vi "Update Palette with Legend.vi"(6 "Control Ref Queue":T1, 8 "error in (no error)":errorcluster, 11 "3D Plot.lvclass":refnum<class "3D Plot.lvclass">) -> (0 "error out":errorcluster, 1 "Ignore the size change?":bool, 3 "3D Plot.lvclass out":refnum<class "3D Plot.lvclass">)   [LabVIEW 2017, in "3D Plot.lvclass"]
uses:
  <vilib>/Math Plots/3D Math Plots/3D Plot/3D Plot/3D Plot.lvclass
  <vilib>/Math Plots/3D Math Plots/3D Plot/Action String/3DMathPlot Ctrl Act Queue.ctl
  <vilib>/Math Plots/3D Math Plots/3D Plot/Action String/3DMathPlot Ctrl Act Cluster.ctl
  <vilib>/Math Plots/3D Math Plots/3D Plot/Action String/3DMathPlot State Class.ctl
  <vilib>/Math Plots/3D Math Plots/3D Plot/3D Plot/3D Plot.lvclass/3D Plot.ctl
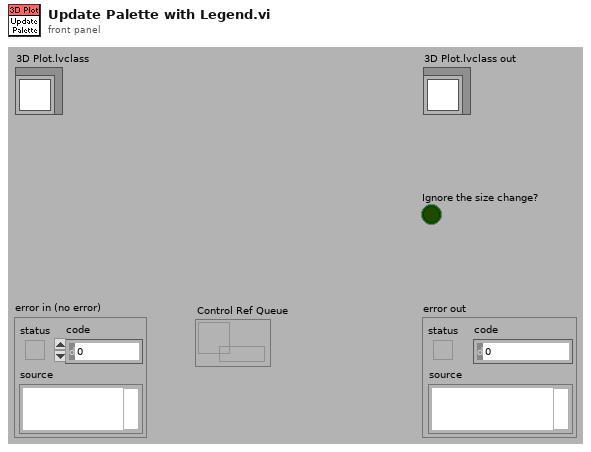
[diagram p1: front panel]
types:
  T1 = typedef "3DMathPlot Ctrl Act Queue.ctl" = refnum<queue>
  T2 = typedef "3DMathPlot Ctrl Act Cluster.ctl" = cluster{"3D Picture Control":refnum<vi>, "Render Window Refnum":refnum<vi>, "XY Graph":refnum<vi>, "Intensity Graph":refnum<vi>, "Color Legend Palette":refnum<vi>, "Projection Palette":refnum<vi>, "XControl  Ref":refnum<vi>, "Facade Ref":refnum<vi>, "Export Image Ref":refnum<vi>, "Clear Data Flag":bool, "Display State Change Class":T3}
  T3 = typedef "3DMathPlot State Class.ctl" = enum16{"Update All Objects (Undo)", "Update Light Object Only", "Update Axis Object Only", "Update Plot Object Only", "Update Cursor Object Only", "Update Axis Plot Cursor Objects", "No Update"}
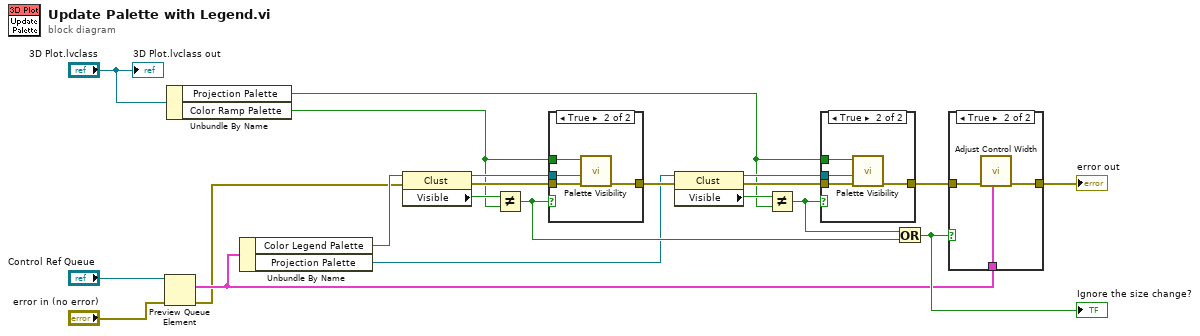
[diagram p0: block diagram]
diagram:
  n1 = Preview Queue Element(queue="Control Ref Queue", error in (no error)="error in (no error)") -> (element=w2:T2, error out=w1:errorcluster)  [unwired: 3 out]
  n2 = Unbundle By Name("3D Plot.lvclass") -> ("Projection Palette"=w5:bool, "Color Ramp Palette"=w6:bool)
  n3 = Unbundle By Name(w2) -> ("Color Legend Palette"=w4:refnum<vi>, "Projection Palette"=w3:refnum<vi>)
  n4 = property class="Clust"(reference=w4, error in=w1) -> (reference out=w15:refnum<vi>, error out=w13:errorcluster, "Visible"=w14:bool)
  n5 = Not Equal?(x=w14, y=w6) -> (x != y?=w8:bool)
  n6 = case shown="True" w8 {
    tunnel: [w22 w26] -> w12
    tunnel: w13 -> [w22 w25]
    tunnel: w15 -> [_ w24]
    tunnel: w6 -> [_ w23]
    frame False {
    }
    frame True {
      n7 = call <vilib>:"Palette Visibility.vi"("error in (no error)"=w25, "Clust Refnum"=w24, "Visible?"=w23) -> ("error out"=w26:errorcluster)  [unwired: 1 in, 7 out]
    }
  }
  n8 = property class="Clust"(reference=w3, error in=w12) -> (reference out=w9:refnum<vi>, error out=w11:errorcluster, "Visible"=w10:bool)
  n9 = Not Equal?(x=w10, y=w5) -> (x != y?=w7:bool)
  n10 = case shown="True" w7 {
    tunnel: w5 -> [_ w31]
    tunnel: w11 -> [w27 w30]
    tunnel: w9 -> [_ w29]
    tunnel: [w27 w28] -> w16
    frame False {
    }
    frame True {
      n11 = call <vilib>:"Palette Visibility.vi"("error in (no error)"=w30, "Clust Refnum"=w29, "Visible?"=w31) -> ("error out"=w28:errorcluster)  [unwired: 1 in, 7 out]
    }
  }
  n12 = Or(x=w7, y=w8) -> (x .or. y?=w20:bool)
  "Ignore the size change?" <- w20
  n13 = case shown="True" w20 {
    tunnel: w16 -> [w32 w35]
    tunnel: [w32 w34] -> w19
    tunnel: w2 -> [_ w33]
    frame False {
    }
    frame True {
      n14 = call <vilib>:"Adjust Control Width.vi"("Control Ref Cluster"=w33, "error in (no error)"=w35) -> ("error out"=w34:errorcluster)  [unwired: 9 out]
    }
  }
  "error out" <- w19
  "3D Plot.lvclass out" <- "3D Plot.lvclass"
